vi "Configure Measurement (Reflection Measurement - Cable).vi"(0 "VISA resource name":refnum<visa-resource-name>, 1 "Attenuation (0 dB/m)":dbl, 5 "Cable Name (5088)":string="5088", 9 "Cable Type (0: S1000)":i32(ring) items=["S1000", "S2000", "S2500", "Custom"], 11 "error in (no error)":errorcluster, 12 "Velocity Factor (1.5)":dbl=1.5) -> (4 "VISA resource name out":refnum<visa-resource-name>, 15 "error out":errorcluster)   [LabVIEW 2022 SP3, in "Agilent N934X Series.lvlib"]
doc: "Configures the cable setting of Reflection Measurement Option.\n\nNotes: \n(1) Option RM7 and TG7 are required to enable the reflection measurement function.\n\n(2) This VI is only applicable for N9321C, N9322C, N9323C, N9324C models"
uses:
  <instrlib>/Agilent N934X Series/Agilent N934X Series.lvlib
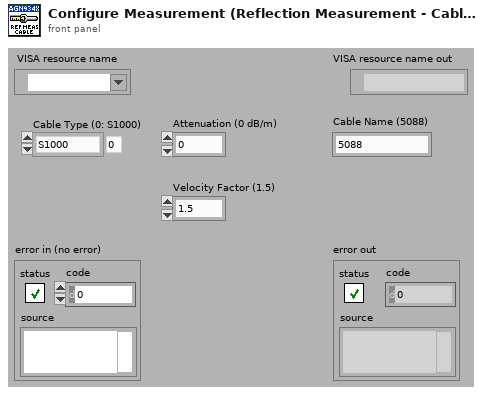
[diagram p1: front panel]
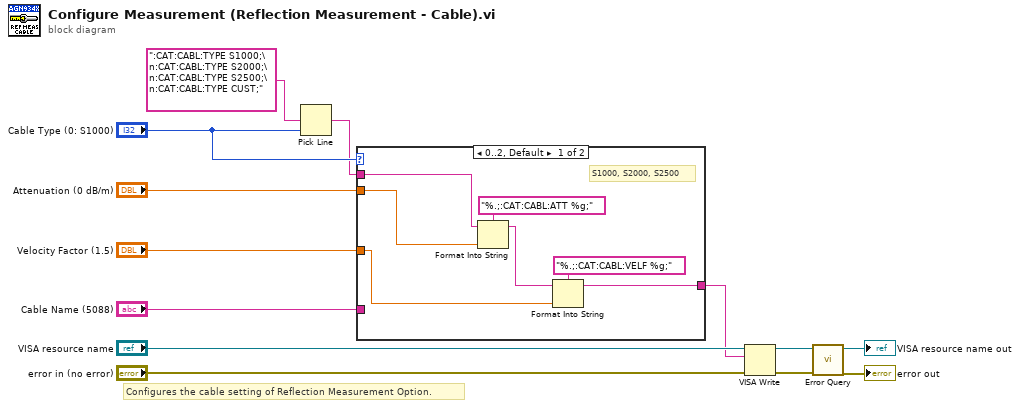
[diagram p0: block diagram]
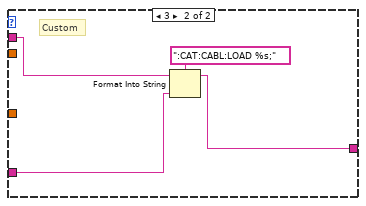
[diagram p2: hidden frame]
diagram:
  # "Configures the cable setting of Reflection Measurement Option."
  n1 = Pick Line(multi-line string=":CAT:CABL:TYPE S1000;\n:CAT:CABL:TYPE S2000;\n:CAT:CABL:TYPE S2500;\n:CAT:CABL:TYPE CUST;", line index="Cable Type (0: S1000)") -> (output string=w2:string)  [unwired: 1 in]
  n2 = case shown="0..2, Default" "Cable Type (0: S1000)" {
    tunnel: "Attenuation (0 dB/m)" -> [w17 _]
    tunnel: "Velocity Factor (1.5)" -> [w16 _]
    tunnel: "Cable Name (5088)" -> [_ w22]
    tunnel: w2 -> [w15 w23]
    tunnel: [w14 w21] -> w1
    frame 0..2, Default {
      # "S1000, S2000, S2500"
      n3 = Format Into String(format string="%.;:CAT:CABL:ATT %g;", initial string=w15, w17) -> (resulting string=w19:string)  [unwired: 1 in, 1 out]
      n4 = Format Into String(format string="%.;:CAT:CABL:VELF %g;", initial string=w19, w16) -> (resulting string=w14:string)  [unwired: 1 in, 1 out]
    }
    frame 3 {
      # "Custom"
      n5 = Format Into String(format string=":CAT:CABL:LOAD %s;", initial string=w23, w22) -> (resulting string=w21:string)  [unwired: 1 in, 1 out]
    }
  }
  n6 = VISA Write(VISA resource name="VISA resource name", write buffer=w1, error in (no error)="error in (no error)") -> (VISA resource name out=w10:refnum<visa-resource-name>, error out=w9:errorcluster)  [unwired: 1 out]
  n7 = call <instrlib>:"Error Query.vi"("error in (no error)"=w9, "VISA resource name"=w10) -> ("error out"=→"error out":errorcluster, "VISA resource name out"=→"VISA resource name out":refnum<visa-resource-name>)  [unwired: 6 in, 2 out]
